vi "write error message.vi"(8 "error in (no error)":errorcluster) -> (3 "element":T1)   [LabVIEW 2015]
uses:
  message/communicator message.lvclass
  message/message.ctl
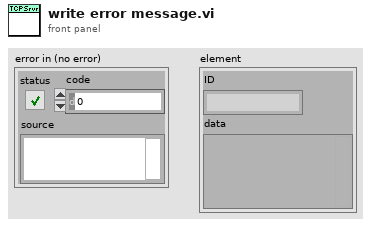
[diagram p1: front panel]
types:
  T1 = typedef "message.ctl" = cluster{"ID":string, "data":variant}
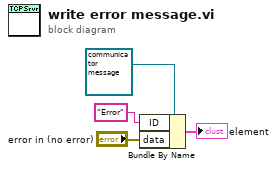
[diagram p0: block diagram]
diagram:
  n1 = Bundle By Name(cluster=refnum<class "communicator message.lvclass"> refnum ("element"), "ID"="Error", "data"="error in (no error)") -> (→"element":cluster{})
